vi "Solid Dilution Control-5.vi"() -> ()   [LabVIEW 2012]
uses:
  <vilib>/DAQmx/read.llb/DAQmx Read (Analog 1D DBL 1Chan NSamp).vi
  <vilib>/Instr/_visa.llb/VISA Configure Serial Port (Instr).vi
  <vilib>/DAQmx/create/channels.llb/DAQmx Create Channel (AI-Strain-Strain Gage).vi
  <vilib>/DAQmx/configure/timing.llb/DAQmx Timing (Sample Clock).vi
  <vilib>/Analysis/baseanly.llb/Mean (DBL).vi
  <vilib>/DAQmx/miscellaneous.llb/DAQmx Fill In Error Info.vi
  <vilib>/Analysis/NI_AALBase.lvlib
panel:
  out "Hydration (g)":dbl
  in  "SIM MASS":dbl=900.0
  in  "real":bool=TRUE
  out "# of Rows Saved":dbl
  out "DAQ Loop":i32=322
  out "SCB Loop":i32=27
  out "Save Loop":i32=19
  out "Main Loop":i32=358
  out "Event Loop":i32
  in  "Tab Control":enum32{"DISPLAY", "CONFIGURE", "Load Cell"}(tab)
  in  "Settings":T1={"ON Settings"={"Enable Dynamic Setpoint?"=TRUE, "Enable Dynamic Dispense Time?"=TRUE, "Enable Drain Rate Functions"=TRUE, "Dispense Sample Time (s)"=0.1, "Dispense Slope Ave"=200, "ON Timeout (sec)"=480.0, "1st Setpoint (% of Target)"=90.0, "2nd Setpoint (% of Target)"=95.0, "3rd Setpoint (% of Target)"=100.0, "Measure Dispense Delay (sec)"=10.0, "Settle Slope Sample Time (s)"=2.0}, "OFF Settings"={"Drain Sample Time (s)"=0.1, "Drain Rate Ave Size"=200, "Drain Rate Limits (± g/sec)"=100.0, "Level Slope Range (± g/sec)"=0.05, "OFF Timeout (sec)"=480.0, "Near SP Slope Level (± g/sec)"=0.005, "Near Setpoint Threshold (%)"=99.0}, "Overshoot Settings"={"Time Limit (s)"=30.0, "Container MAX (g)"=1500.0, "Max FILL Slope (+/- g/sec)"=100.0, "% Overshot to Enable (>)"=3.0}, "FILL Timeout (s)"=300.0, "Full \nSettle Time (s)"=30.0, "Pre-Hydrate \nSpray Time (s)"=10.0, "Pre-Hydrate \nWait Time (s)"=30.0} {"OFF Settings"."Near SP Slope Level (± g/sec)" format="%.3g"; "OFF Settings"."Level Slope Range (± g/sec)" format="%.3g"}
  out "Values":T2 {"Drain Time (s)" format="%.2f"; "Drain Rate (g/sec)" format="%.2f"; "Spray Mass Loss (g)" format="%.2f"; "Time Elapsed (s)" format="%.2f"; "Time Target (s)" format="%.2f"; "Dynamic Setpoint (g)" format="%.2f"; "Static Setpoint (g)" format="%.2f"; "Grams to Setpoint" format="%.2f"; "Adjusted Mass (g)" format="%.2f"; "Dispense Rate (g/sec)" format="%.2f"; "Fill Mass (g)" format="%.2f"; "Fill Rate (g/sec)" format="%.2f"}
  in  "Tare":bool
  in  "Settings Button":bool
  in  "START Dispense":bool
  in  "STOP Dispense":bool
  in  "Fill Setpoint (g)":dbl=750.0
  in  "Dispense Setpoint (%)":dbl=10.0
  out "Mass Chart":T3(graph)={"Grams (SCB)"=0.0, "Fill Target"=900.0, "Dispense Target"=0.0}
  out "Signals":T4={"Dispense"=FALSE, "Fill"=FALSE, "Spray"=FALSE, "Drain"=TRUE, "Complete"=FALSE, "Fill Error"=FALSE, "Dispense Error"=FALSE, "Fill Timeout"=FALSE, "Dispense Timeout"=FALSE}
  in  "Overshoot Adjust?":bool
  out "Dispense Mode":T5(ring)
  out "Product Mass (g)":dbl
  in  "Save Interval (s)":dbl=1.0
  in  "Write/Read Wait (ms)":u32=100
  in  "Event Loop Wait (ms)":i32=5000
  in  "File Path Input":path
  out "SCB Error":errorcluster={"status"=TRUE, "code"=-1073807343, "source"="Property Node (arg 1) in Read SCB via ESP (SubVI).vi->Solid Dilution Control-4.vi"}
  out "SCB Output":T6
  in  "SCB COM Port":refnum<visa-resource-name>="COM5"
  in  "SCB Baud Rate":u32=9600
  in  "DAQ COM Port":refnum<visa-resource-name>="COM4"
  in  "DAQ Baud Rate":u32=115200
  in  "Minimum Wait (ms)":u32=100
  in  "Module Address":i32=1
  in  "Relay Control":T7
  out "DAQ Com Error":errorcluster={"status"=TRUE, "code"=-1073807343, "source"="Property Node (arg 1) in VISA Configure Serial Port (Instr).vi->Solid Dilution Control-4.vi"}
  out "DAQ Error":errorcluster={"status"=TRUE, "code"=-1073807343, "source"="VISA Write in 7067 Relay Module (SubVI).vi->Solid Dilution Control-4.vi"}
  out "Relays Active?":bool
  out "SCB Com Error":errorcluster={"status"=TRUE, "code"=-1073807343, "source"="Property Node (arg 1) in VISA Configure Serial Port (Instr).vi->Solid Dilution Control-4.vi"}
  out "Save Error":errorcluster caption="Error Output"
  out "Weight (Grams)":dbl format="%.2f"
  out "Product Values":T8
  out "CDAQ Array":dbl[](graph)
  out "Grams (Tedea 1040 CDAQ)":dbl[](graph)
  in  "Minimum Value":dbl=-0.001 format="%0.3f"
  in  "Maximum Value":dbl=0.001 format="%0.3f"
  in  "CDAQ Channel":tag="Dev2/ai1"
  out "CDAQ Error":errorcluster={"status"=TRUE, "code"=-201003, "source"="DAQmx Create Channel (AI-Strain-Strain Gage).vi:1<append>\n<B>Device Specified: </B>Dev2\n\n<B>Task Name: </B>_unnamedTask<0>"}
  out "Raw Ave (Tedea 1040 CDAQ)":dbl=nan
  in  "Y LO (g)":dbl
  in  "Y HI (g)":dbl=5000.0
  in  "Set HI":bool
  in  "Set LO":bool
  out "CDAQ Sample Size":i32
  in  "CDAQ Wait (ms)":u32=100
  in  "CDAQ RATE":dbl=1000.0 caption="Rate" format="%0.2f"
  out "CDAQ Loop":i32
  in  "LO":dbl
  in  "HI":dbl
  out "Array":dbl[](array[numeric])
  in  "Save (Enable/Signal)":bool
  in  "STOP PROGRAM":bool=TRUE
  # "SOLID DILUTION CONTROL SYSTEM"
  # "Program Last Updated 2/23/10"
  # "SAVE\nENABLE"
  # "Blake Otting - Systems Engineering Lab - 2009 /2010"
  # "DISPENSE CONTROL"
  # "ONLY ADJUST\nBOLD VALUES!"
  # "GRAMS"
  # "SIGNAL"
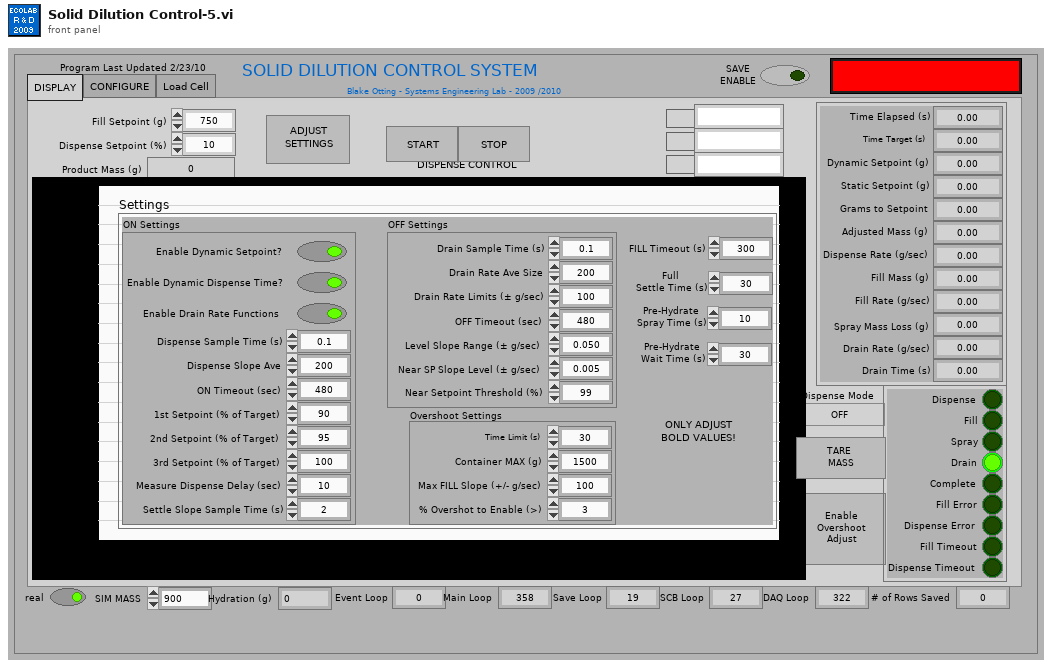
[diagram p1: front panel]
types:
  T1 = cluster{"ON Settings":cluster{"Enable Dynamic Setpoint?":bool, "Enable Dynamic Dispense Time?":bool, "Enable Drain Rate Functions":bool, "Dispense Sample Time (s)":dbl, "Dispense Slope Ave":i32, "ON Timeout (sec)":dbl, "1st Setpoint (% of Target)":dbl, "2nd Setpoint (% of Target)":dbl, "3rd Setpoint (% of Target)":dbl, "Measure Dispense Delay (sec)":dbl, "Settle Slope Sample Time (s)":dbl}, "OFF Settings":cluster{"Drain Sample Time (s)":dbl, "Drain Rate Ave Size":i32, "Drain Rate Limits (± g/sec)":dbl, "Level Slope Range (± g/sec)":dbl, "OFF Timeout (sec)":dbl, "Near SP Slope Level (± g/sec)":dbl, "Near Setpoint Threshold (%)":dbl}, "Overshoot Settings":cluster{"Time Limit (s)":dbl, "Container MAX (g)":dbl, "Max FILL Slope (+/- g/sec)":dbl, "% Overshot to Enable (>)":dbl}, "FILL Timeout (s)":dbl, "Full \nSettle Time (s)":dbl, "Pre-Hydrate \nSpray Time (s)":dbl, "Pre-Hydrate \nWait Time (s)":dbl}
  T2 = cluster{"Time Elapsed (s)":dbl, "Time Target (s)":dbl, "Dynamic Setpoint (g)":dbl, "Static Setpoint (g)":dbl, "Grams to Setpoint":dbl, "Adjusted Mass (g)":dbl, "Dispense Rate (g/sec)":dbl, "Fill Mass (g)":dbl, "Fill Rate (g/sec)":dbl, "Spray Mass Loss (g)":dbl, "Drain Rate (g/sec)":dbl, "Drain Time (s)":dbl}
  T3 = cluster{"Grams (SCB)":dbl, "Fill Target":dbl, "Dispense Target":dbl}
  T4 = cluster{"Dispense":bool, "Fill":bool, "Spray":bool, "Drain":bool, "Complete":bool, "Fill Error":bool, "Dispense Error":bool, "Fill Timeout":bool, "Dispense Timeout":bool}
  T5 = enum16{"OFF", "INITIAL", "FILL", "DISPENSE", "ADJUST"}
  T6 = cluster{"Sequence #":string, "Weight":string, "Status":string, "CRC & EOT":string}
  T7 = cluster{"Master (All Relays)":bool, "Relay1":bool, "Relay2":bool, "Relay3":bool, "Relay4":bool, "Relay5":bool, "Relay6":bool, "Relay7":bool}
  T8 = cluster{"Drain Delta":dbl, "Spray Delta":dbl, "Dispense Delta":dbl}
  T9 = cluster{"Grams (SCB)":dbl, "Fill Target":dbl, "Dispense Target":dbl}[]
  T10 = cluster{"Row Limit":dbl, "Title Block?":bool, "Column Headers?":bool, "Include Time & Elapsed Time?":bool, "Default File Name":string, "Data Array Precision":i16, "Include Comments?":bool, "New File Daily?":bool}
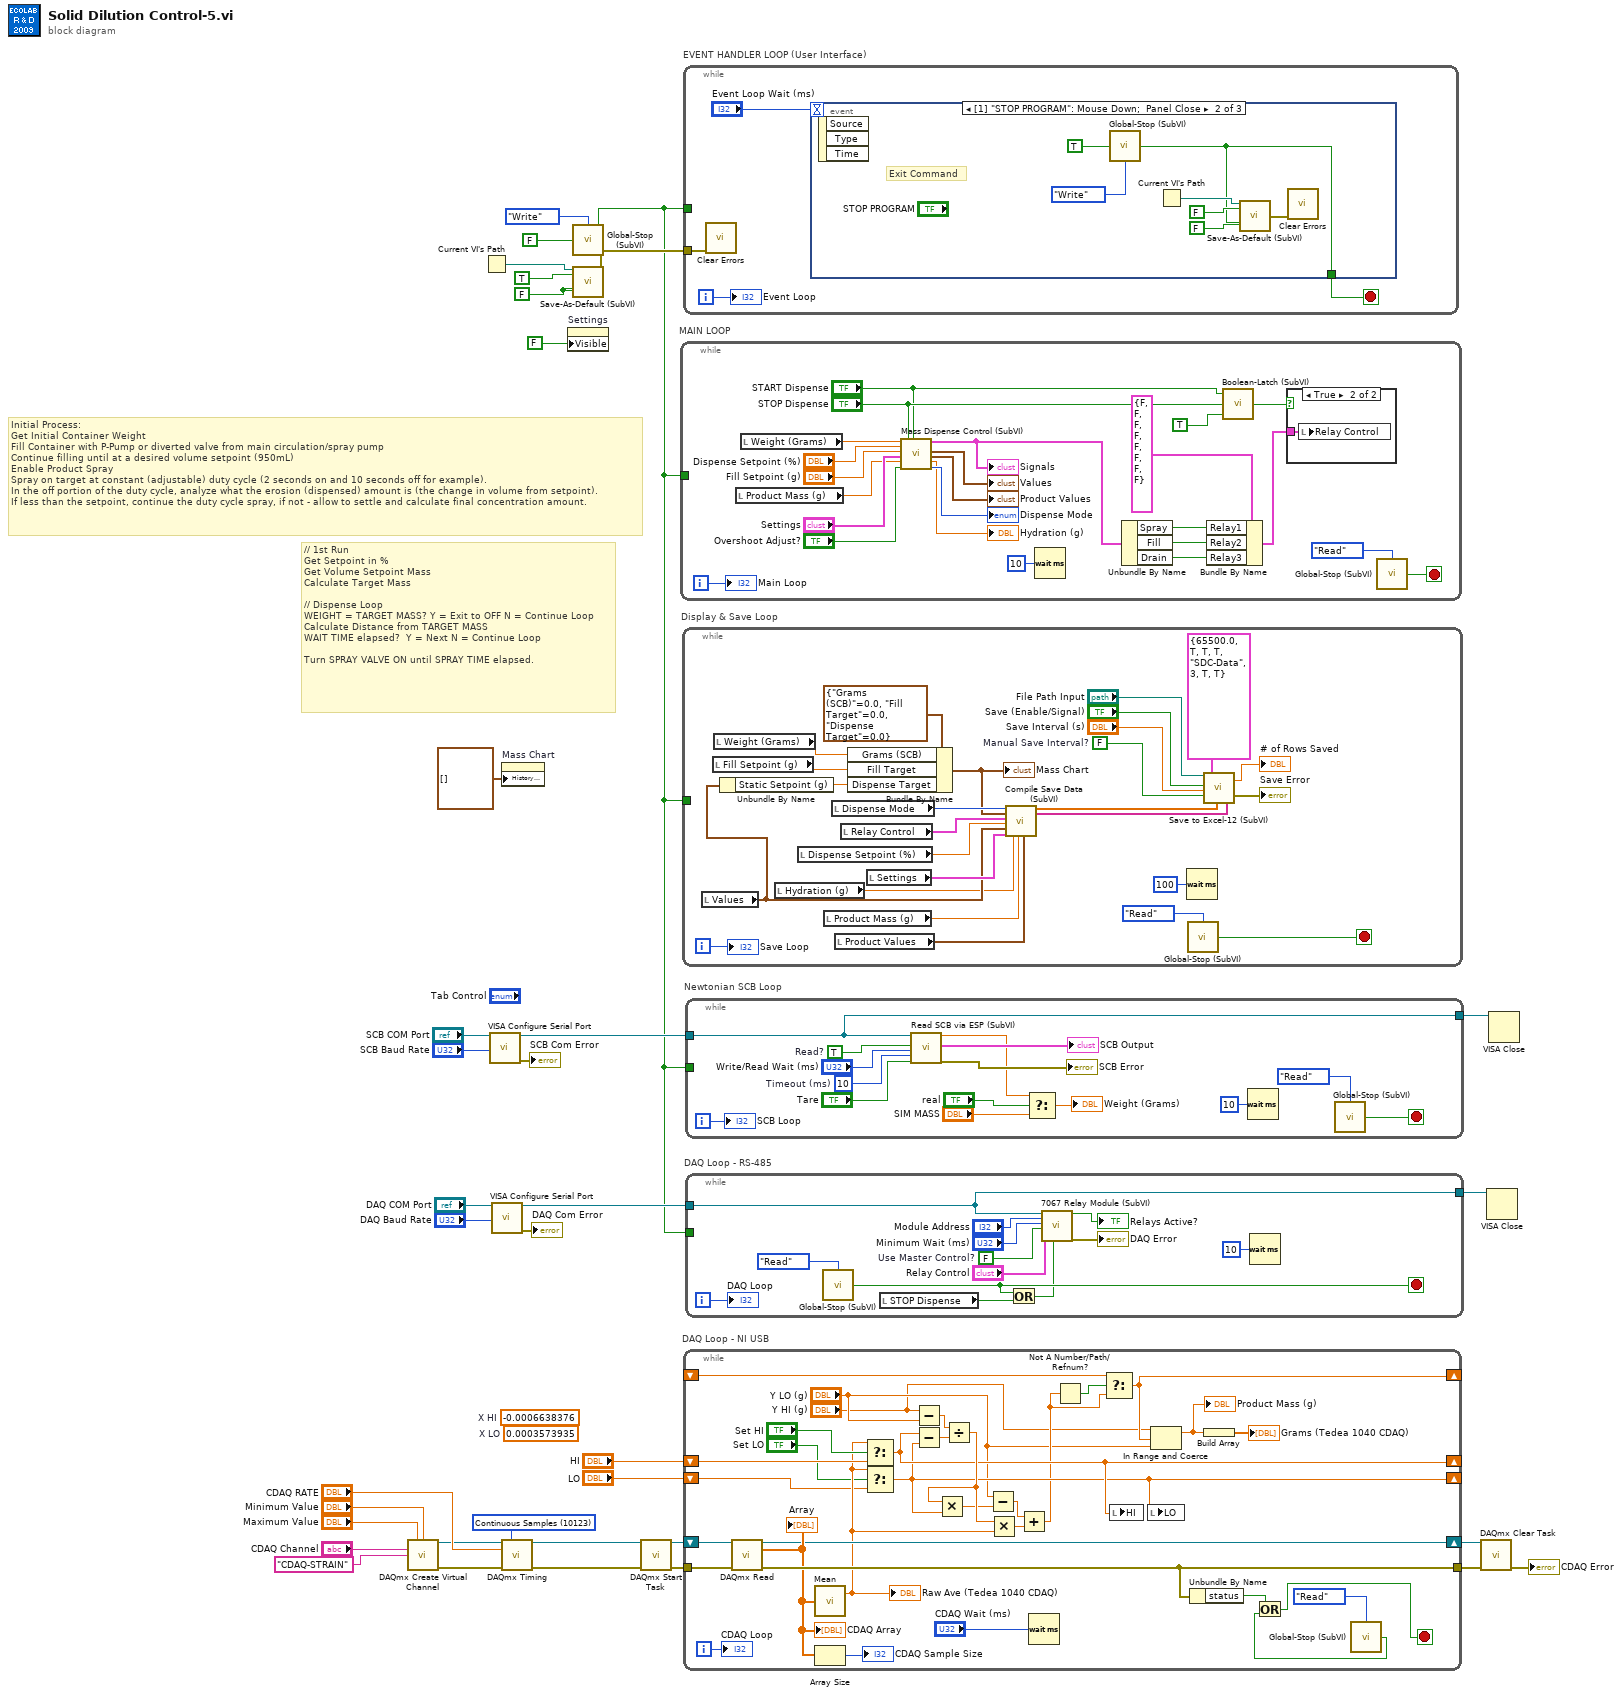
[diagram p0: block diagram]
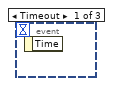
[diagram p3: hidden frame]
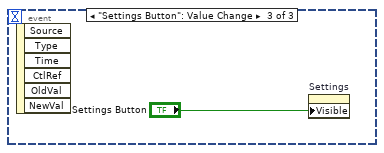
[diagram p4: hidden frame]
diagram:
  (unwired) 0.0003573935  # X LO
  (unwired) -0.0006638376  # X HI
  w17 = 10123 items=["Finite Samples"=10178, "Continuous Samples"=10123] ("sample mode")
  w22 = FALSE ("Save Settings")
  # "// 1st Run\nGet Setpoint in %\nGet Volume Setpoint Mass\nCalculate Target Mass\n\n// Dispense Loop\nWEIGHT = TARGET MASS? Y = Exit to OFF N = Continue Loop\nCalculate Distance from TARGET MASS\nWAIT TIME elapsed?  Y = Next N = Continue Loop\n\nTurn SPRAY VALVE ON until SPRAY TIME elapsed."
  # "Initial Process:\nGet Initial Container Weight\nFill Container with P-Pump or diverted valve from main circulation/spray pump\nContinue filling until at a desired volume setpoint (950mL)\nEnable Product Spray\nSpray on target at constant (adjustable) duty cycle (2 seconds on and 10 seconds off for example).\nIn the off portion of the duty cycle, analyze what the erosion (dispensed) amount is (the change in volume from setpoint).  \nIf less than the setpoint, continue the duty cycle spray, if not - allow to settle and calculate final concentration amount."
  n1 = call-poly <vilib>:"DAQmx Create Virtual Channel.vi"("maximum value"="Maximum Value", "minimum value"="Minimum Value", "physical channels"="CDAQ Channel", "name to assign"="CDAQ-STRAIN") -> ("task out"=w14:refnum<k21>, "error out"=w15:errorcluster)  [unwired: 8 in, 2 out]
  n2 = Current VI's Path() -> (path=w24:path)
  n3 = call-poly "VISA Configure Serial Port"("VISA resource name"="SCB COM Port", "baud rate (9600)"="SCB Baud Rate") -> ("VISA resource name out"=w29:refnum<visa-resource-name>, "error out"=→"SCB Com Error":errorcluster)  [unwired: 4 in, 8 out]
  n4 = call-poly "VISA Configure Serial Port"("VISA resource name"="DAQ COM Port", "baud rate (9600)"="DAQ Baud Rate") -> ("VISA resource name out"=w34:refnum<visa-resource-name>, "error out"=→"DAQ Com Error":errorcluster)  [unwired: 4 in, 8 out]
  n5 = property on="Mass Chart" class="WFChart (strict)"("History Data"=T9 []) -> ()  [unwired: 2 in, 2 out]
  n6 = call-poly <vilib>:"DAQmx Timing.vi"("task/channels in"=w14, "sample mode"=w17, "rate"="CDAQ RATE", "error in"=w15) -> ("task out"=w9:refnum<k21>, "error out"=w7:errorcluster)  [unwired: 3 in, 7 out]
  n7 = property on="Settings" class="Clust (strict)"("Visible"=FALSE) -> ()  [unwired: 2 in, 2 out]
  n8 = call "Global-Stop (SubVI).vi"("Mode (Read)"=enum16{"Read", "Write"}."Write", "IN"=FALSE) -> ("OUT"=w18:bool)  [unwired: 2 out]
  n9 = call "Save-As-Default (SubVI).vi"("Current VI's Path"=w24, "Load Settings"=TRUE, "Save Settings"=w22, "Save and Exit"=w22) -> ("Save as Default Error"=w21:errorcluster)  [unwired: 9 in, 2 out]
  n10 = call <vilib>:"DAQmx Start Task.vi"("task/channels in"=w9, "error in"=w7) -> ("task out"=w8:refnum<k21>, "error out"=w6:errorcluster)  [unwired: 12 out]
  n11 = while "MAIN LOOP" {
    tunnel: w18 -> [_]
    i -> [w53]
    stop <- w56 stop-if-true
    n12 = local read "Product Mass (g)"() -> (w39:dbl)
    n13 = local read "Weight (Grams)"() -> (w43:dbl)
    n14 = call "Mass Dispense Control (SubVI).vi"("Weight (Grams)"=w43, "Dispense Setpoint (%)"="Dispense Setpoint (%)", "Fill Setpoint (g)"="Fill Setpoint (g)", "Settings"="Settings", "Product Weight (g)"=w39, "Overshoot Adjust?"="Overshoot Adjust?", "STOP Dispense"="STOP Dispense", "START Dispense"="START Dispense") -> ("Signals"=w44:T4, "Values"=→"Values":T2, "Product Values"=→"Product Values":T8, "Hydration (g)"=→"Hydration (g)":dbl, "Dispense Mode"=→"Dispense Mode":T5)  [unwired: 7 out]
    "Signals" <- w44
    n15 = Wait (ms)(milliseconds to wait=u32 10) -> ()  [unwired: 1 out]
    n16 = Unbundle By Name(w44) -> ("Spray"=w52:bool, "Fill"=w51:bool, "Drain"=w57:bool)
    n17 = Bundle By Name(cluster=T7 {"Master (All Relays)"=FALSE, "Relay1"=FALSE, "Relay2"=FALSE, "Relay3"=FALSE, "Relay4"=FALSE, "Relay5"=FALSE, "Relay6"=FALSE, "Relay7"=FALSE} ("Relay Control"), "Relay1"=w52, "Relay2"=w51, "Relay3"=w57) -> (w54:T7)
    n18 = call "Boolean-Latch (SubVI).vi"("Reset on First Call (T)"=TRUE, "Reset"="STOP Dispense", "Trigger (Input)"="START Dispense") -> ("Latched? (Output)"=w55:bool)
    n19 = case shown="True" w55 {
      tunnel: w54 -> [_ w61]
      frame False {
      }
      frame True {
        n20 = local write "Relay Control"(w61) -> ()
      }
    }
    n21 = call "Global-Stop (SubVI).vi"("Mode (Read)"=enum16{"Read", "Write"}."Read") -> ("OUT"=w56:bool)  [unwired: 1 in, 2 out]
    "Main Loop" <- w53
  }
  n22 = while "Display & Save Loop" {
    tunnel: w18 -> [_]
    i -> [w78]
    stop <- w85 stop-if-true
    w80 = FALSE  # Manual Save Interval?
    n23 = local read "Values"() -> (w67:T2)
    n24 = local read "Fill Setpoint (g)"() -> (w69:dbl)
    n25 = local read "Weight (Grams)"() -> (w70:dbl)
    n26 = Unbundle By Name(w67) -> ("Static Setpoint (g)"=w76:dbl)
    n27 = local read "Hydration (g)"() -> (w63:dbl)
    n28 = local read "Dispense Setpoint (%)"() -> (w72:dbl)
    n29 = local read "Product Mass (g)"() -> (w65:dbl)
    n30 = local read "Dispense Mode"() -> (w68:T5)
    n31 = local read "Product Values"() -> (w64:T8)
    n32 = local read "Relay Control"() -> (w73:T7)
    n33 = Bundle By Name(cluster=T3 {"Grams (SCB)"=0.0, "Fill Target"=0.0, "Dispense Target"=0.0} ("Conductivity"), "Grams (SCB)"=w70, "Fill Target"=w69, "Dispense Target"=w76) -> (w66:T3)
    "Mass Chart" <- w66
    n34 = local read "Settings"() -> (w71:T1)
    n35 = call "Compile Save Data (SubVI).vi"("Dispense Mode"=w68, "Mass Chart"=w66, "Relay Control"=w73, "Dispense Setpoint (%)"=w72, "Values"=w67, "Settings"=w71, "Hydration (g)"=w63, "Product Mass (g)"=w65, "Product Values"=w64) -> ("Data Array Output"=w74:dbl[], "Column Header Text Array"=w75:string[])  [unwired: 9 out]
    n36 = Wait (ms)(milliseconds to wait=u32 100) -> ()  [unwired: 1 out]
    n37 = call "Global-Stop (SubVI).vi"("Mode (Read)"=enum16{"Read", "Write"}."Read") -> ("OUT"=w85:bool)  [unwired: 1 in, 2 out]
    n38 = call "Save to Excel-12 (SubVI).vi"("File Path Input"="File Path Input", "Save (Enable/Signal)"="Save (Enable/Signal)", "Save Interval (s)"="Save Interval (s)", "Manual Save Interval?"=w80, "File Configuration"=T10 {"Row Limit"=65500.0, "Title Block?"=TRUE, "Column Headers?"=TRUE, "Include Time & Elapsed Time?"=TRUE, "Default File Name"="SDC-Data", "Data Array Precision"=3, "Include Comments?"=TRUE, "New File Daily?"=TRUE}, "Data Array (Row)"=w74, "Column Header Text Array"=w75) -> ("# of Rows Saved"=→"# of Rows Saved":dbl, "Error Output"=→"Save Error":errorcluster)  [unwired: 5 in, 6 out]
    "Save Loop" <- w78
  }
  n39 = while "EVENT HANDLER LOOP (User Interface)" {
    tunnel: w18 -> [_]
    tunnel: w21 -> [w89]
    i -> [w88]
    stop <- w91 stop-if-true
    n40 = call <vilib>:"Clear Errors.vi"("error in (no error)"=w89) -> ()  [unwired: 7 out]
    n41 = event shown="[1] \"STOP PROGRAM\": Mouse Down;  Panel Close" {
      selector: _ -> [_ _ _]
      dyn-events: _ -> [_ _ _]
      timeout: "Event Loop Wait (ms)" -> [_ _ _]
      tunnel: [_ w93 _] -> w91
      event Timeout {
        n42 = event-data() -> ()  [unwired: 2 out]
      }
      event "STOP PROGRAM": Mouse Down; Panel Close {
        # "Exit Command"
        n43 = event-data() -> ()  [unwired: 4 out]
        n44 = call "Global-Stop (SubVI).vi"("Mode (Read)"=enum16{"Read", "Write"}."Write", "IN"=TRUE) -> ("OUT"=w93:bool)  [unwired: 2 out]
        n45 = Current VI's Path() -> (path=w95:path)
        n46 = call "Save-As-Default (SubVI).vi"("Current VI's Path"=w95, "Load Settings"=FALSE, "Save Settings"=w93, "Save and Exit"=FALSE ("Save Settings")) -> ("Save as Default Error"=w92:errorcluster)  [unwired: 9 in, 2 out]
        n47 = call <vilib>:"Clear Errors.vi"("error in (no error)"=w92) -> ()  [unwired: 7 out]
      }
      event "Settings Button": Value Change {
        n48 = event-data() -> ()  [unwired: 7 out]
        n49 = property on="Settings" class="Clust (strict)"("Visible"="Settings Button") -> ()  [unwired: 2 in, 2 out]
      }
    }
    "Event Loop" <- w88
  }
  n50 = while "DAQ Loop - NI USB" {
    tunnel: w6 -> [w119]
    tunnel: [w118] -> w5
    shift-right: [w115] -> w3
    shift-left: w8 -> [w120]
    shift-right: [w108] -> _
    shift-left: "HI" -> [w113]
    shift-right: [w107] -> _
    shift-left: "LO" -> [w110]
    shift-right: [w102] -> _
    shift-left: _ -> [w105]
    i -> [w109]
    stop <- w121 stop-if-true
    n51 = call-poly <vilib>:"DAQmx Read.vi"("task/channels in"=w120, "error in"=w119) -> ("task out"=w115:refnum<k21>, "data"=w116:dbl[], "error out"=w118:errorcluster)  [unwired: 1 in, 10 out]
    "CDAQ Array" <- w116
    "Array" <- w116
    n52 = call-poly <vilib>:"Mean.vi"("X"=w116) -> ("mean"=w112:dbl)  [unwired: 1 out]
    "Raw Ave (Tedea 1040 CDAQ)" <- w112
    n53 = Array Size(array=w116) -> (size(s)=→"CDAQ Sample Size":i32)
    n54 = Select(t=w112, s="Set HI", f=w113) -> (s? t:f=w108:dbl)
    n55 = Select(t=w112, s="Set LO", f=w110) -> (s? t:f=w107:dbl)
    n56 = Subtract(x="Y HI (g)", y="Y LO (g)") -> (x-y=w124:dbl)
    n57 = Subtract(x=w108, y=w107) -> (x-y=w125:dbl)
    n58 = Divide(x=w124, y=w125) -> (x/y=w127:dbl)
    n59 = Multiply(x=w127, y=w107) -> (x*y=w126:dbl)
    n60 = Subtract(x="Y LO (g)", y=w126) -> (x-y=w128:dbl)
    n61 = Multiply(x=w127, y=w112) -> (x*y=w129:dbl)
    n62 = Add(x=w128, y=w129) -> (x+y=w104:dbl)
    n63 = Wait (ms)(milliseconds to wait="CDAQ Wait (ms)") -> ()  [unwired: 1 out]
    n64 = Not A Number/Path/Refnum?(number/path/refnum=w104) -> (NaN/Path/Refnum?=w106:bool)
    n65 = Select(t=w105, s=w106, f=w104) -> (s? t:f=w102:dbl)
    n66 = local write "HI"(w108) -> ()
    n67 = local write "LO"(w107) -> ()
    n68 = In Range and Coerce(upper limit="Y HI (g)", x=w102, lower limit="Y LO (g)") -> (coerced(x)=w100:dbl)  [unwired: 1 out]
    "Product Mass (g)" <- w100
    n69 = Unbundle By Name(w118) -> ("status"=w123:bool)
    n70 = Build Array(w100) -> (→"Grams (Tedea 1040 CDAQ)":dbl[])
    n71 = call "Global-Stop (SubVI).vi"("Mode (Read)"=enum16{"Read", "Write"}."Read") -> ("OUT"=w122:bool)  [unwired: 1 in, 2 out]
    n72 = Or(x=w123, y=w122) -> (x .or. y?=w121:bool)
    "CDAQ Loop" <- w109
  }
  n73 = while "Newtonian SCB Loop" {
    tunnel: w29 -> [w139]
    tunnel: [w139] -> w26
    tunnel: w18 -> [_]
    i -> [w137]
    stop <- w141 stop-if-true
    w147 = TRUE  # Read?
    w145 = u32 10  # Timeout (ms)
    n74 = call "Read SCB via ESP (SubVI).vi"("COM Port Input"=w139, "Manual Write Command"=w147, "Write/Read Wait (ms)"="Write/Read Wait (ms)", "Timeout (ms)"=w145, "Tare"="Tare") -> ("Weight (Grams)"=w135:dbl, "SCB Output"=→"SCB Output":T6, "Error Output"=→"SCB Error":errorcluster)  [unwired: 12 out]
    n75 = Select(t=w135, s="real", f="SIM MASS") -> (s? t:f=→"Weight (Grams)":dbl)
    n76 = Wait (ms)(milliseconds to wait=u32 10) -> ()  [unwired: 1 out]
    n77 = call "Global-Stop (SubVI).vi"("Mode (Read)"=enum16{"Read", "Write"}."Read") -> ("OUT"=w141:bool)  [unwired: 1 in, 2 out]
    "SCB Loop" <- w137
  }
  n78 = while "DAQ Loop - RS-485" {
    tunnel: w34 -> [w152]
    tunnel: [w152] -> w25
    tunnel: w18 -> [_]
    i -> [w151]
    stop <- w149 stop-if-true
    w158 = FALSE  # Use Master Control?
    n79 = call "Global-Stop (SubVI).vi"("Mode (Read)"=enum16{"Read", "Write"}."Read") -> ("OUT"=w149:bool)  [unwired: 1 in, 2 out]
    n80 = local read "STOP Dispense"() -> (w150:bool)
    n81 = Or(x=w149, y=w150) -> (x .or. y?=w148:bool)
    n82 = call "7067 Relay Module (SubVI).vi"("COM Port"=w152, "Module Address"="Module Address", "Minimum Wait (ms)"="Minimum Wait (ms)", "Use Master Control?"=w158, "Relay Control"="Relay Control", "E-STOP (ALL OFF)"=w148) -> ("Relays Active?"=→"Relays Active?":bool, "Error Output"=→"DAQ Error":errorcluster)  [unwired: 12 out]
    n83 = Wait (ms)(milliseconds to wait=u32 10) -> ()  [unwired: 1 out]
    "DAQ Loop" <- w151
  }
  n84 = call <vilib>:"DAQmx Clear Task.vi"("task in"=w3, "error in"=w5) -> ("error out"=→"CDAQ Error":errorcluster)  [unwired: 13 out]
  n85 = VISA Close(VISA resource name=w25) -> ()  [unwired: 1 in, 1 out]
  n86 = VISA Close(VISA resource name=w26) -> ()  [unwired: 1 in, 1 out]
